vi "LaserCal-Clear Voltages.vi"(11 "error in (no error)":errorcluster) -> (15 "error out":errorcluster)   [LabVIEW 2015]
panel:
  in  "T (s)":dbl=0.25
  in  "Fs (Hz)":dbl=100000.0
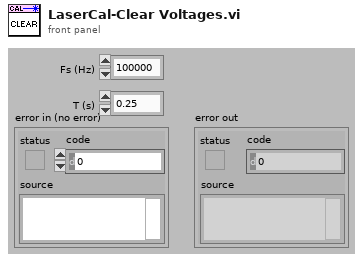
[diagram p1: front panel]
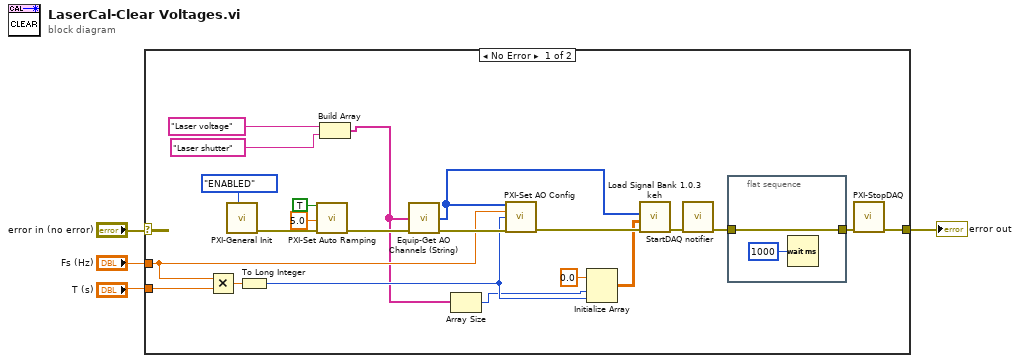
[diagram p0: block diagram]
diagram:
  n1 = case shown="No Error" "error in (no error)" {
    selector: "error in (no error)" -> [_ w29]
    tunnel: [w5 w29] -> w3
    tunnel: "Fs (Hz)" -> [w22 _]
    tunnel: "T (s)" -> [w24 _]
    frame No Error {
      n2 = Multiply(x=w22, y=w24) -> (x*y=w23:dbl)
      n3 = call "PXI-General Init.vi"("Double Buffer Mode"=enum32{"OFF", "ENABLED", "FORCED"}."ENABLED") -> ("error out"=w19:errorcluster)  [unwired: 10 in]
      n4 = To Long Integer(number=w23) -> (32bit integer=w12:i32)
      n5 = call "PXI-Set Auto Ramping.vi"("Auto ramp?"=TRUE, "Ramp duration (ms)"=5.0, "error in (no error)"=w19) -> ("error out"=w18:errorcluster)  [unwired: 12 in]
      n6 = Build Array("Laser voltage" ("String"), "Laser shutter" ("String")) -> (w9:string[])
      n7 = call "Equip-Get AO Channels (String).vi"("Channel Names"=w9, "error in (no error)"=w18) -> ("AO Channels"=w13:i32[], "error out"=w25:errorcluster)  [unwired: 12 in]
      n8 = Array Size(array=w9) -> (size(s)=w8:i32)
      n9 = call "PXI-Set AO Config.vi"("AO Channels"=w13, "Sampling Rate (Hz)"=w22, "Buffer Size"=w12, "error in (no error)"=w25) -> ("error out"=w15:errorcluster)  [unwired: 11 in]
      n10 = Initialize Array(0.0 ("element"), w8, w12) -> (w10:dbl[][])
      n11 = call "Load Signal Bank 1.0.3 keh.vi"("error in (no error)"=w15, "Input array"=w10, "Active AO Array"=w13) -> ("error out"=w14:errorcluster)  [unwired: 6 in, 2 out]
      n12 = call "StartDAQ notifier.vi"("error in (no error)"=w14) -> ("error out"=w6:errorcluster)  [unwired: 6 in]
      n13 = flat-sequence {
        tunnel: [w27] -> w7
        tunnel: w6 -> [w27]
        frame #0 {
          n14 = Wait (ms)(milliseconds to wait=u32 1000) -> ()  [unwired: 1 out]
        }
      }
      n15 = call "PXI-StopDAQ.vi"("error in (no error)"=w7) -> ("error out"=w5:errorcluster)  [unwired: 6 in]
    }
    frame Error {
    }
  }
  "error out" <- w3
